vi "REPORT_CFG_prepare_header_for_csv.vi"(11 "REPORT_CFG_all_info":T1) -> (3 "report_header":string[][](array[string]))   [LabVIEW 2019]
uses:
  typedef/REPORT_CFG_all_info.ctl
  typedef/REPORT_CFG_types.ctl
  _misc/AULocalize/SubVIs/Get Localized Phrase Compact Interface 1D.vi
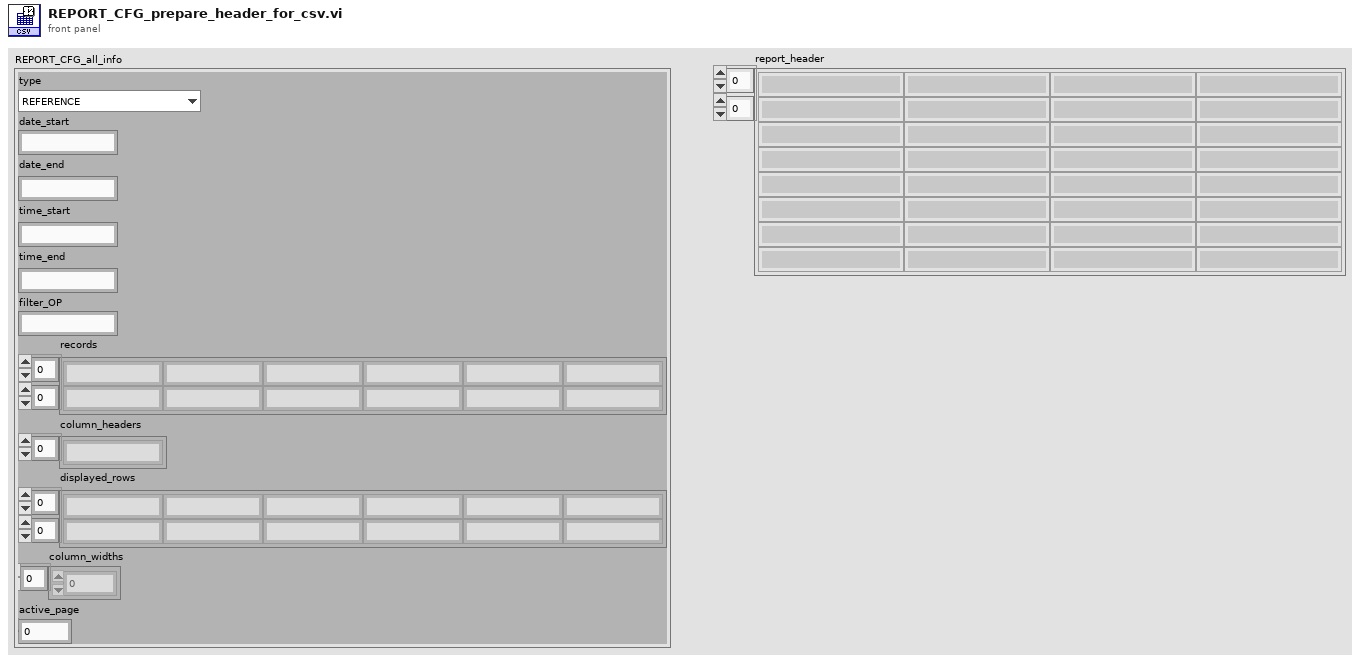
[diagram p1: front panel]
types:
  T1 = typedef "REPORT_CFG_all_info.ctl" = cluster{"type":T2, "date_start":string, "date_end":string, "time_start":string, "time_end":string, "filter_OP":string, "records":string[][], "column_headers":string[], "displayed_rows":string[][], "column_widths":i16[], "active_page":i32}
  T2 = typedef "REPORT_CFG_types.ctl" = enum16{"REFERENCE", "ARCHIVISATION", "USERS"}
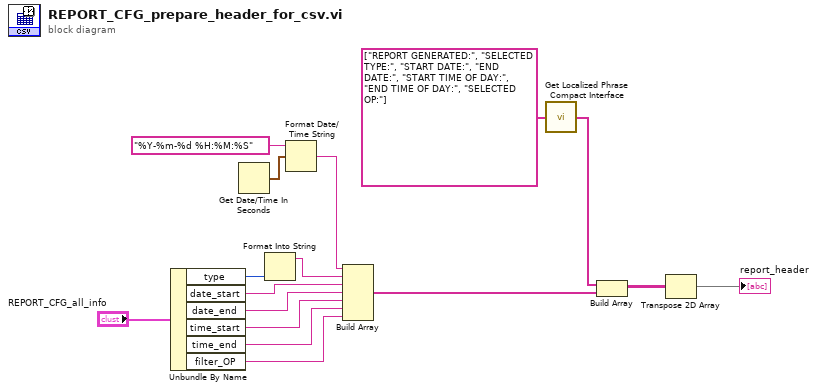
[diagram p0: block diagram]
diagram:
  n1 = Unbundle By Name("REPORT_CFG_all_info") -> ("type"=w3:T2, "date_start"=w10:string, "date_end"=w9:string, "time_start"=w6:string, "time_end"=w5:string, "filter_OP"=w4:string)
  n2 = Get Date/Time In Seconds() -> (seconds since 1Jan1904=w15:timestamp)
  n3 = Format Into String(w3) -> (resulting string=w2:string)  [unwired: 3 in, 1 out]
  n4 = Format Date/Time String(time format string (%c)="%Y-%m-%d %H:%M:%S", seconds (now)=w15) -> (date/time string=w8:string)  [unwired: 1 in]
  n5 = Build Array(w8, w2, w10, w9, w6, w5, w4) -> (w11:string[])
  n6 = call-poly "Get Localized Phrase Compact Interface.vi"("Key"=string[] ["REPORT GENERATED:", "SELECTED TYPE:", "START DATE:", "END DATE:", "START TIME OF DAY:", "END TIME OF DAY:", "SELECTED OP:"]) -> ("Translated Phrase"=w1:string[])
  n7 = Build Array(w1, w11) -> (w14:string[][])
  n8 = Transpose 2D Array(2D array=w14) -> (transposed array=→"report_header":string[][])
